vi "CalculerPolynome.vi"(6 "Résidu [in]":dbl, 8 "e3 [in]":dbl, 9 "Meilleure poly [in]":dbl[](array[numeric]), 10 "Y":dbl[](array[numeric]), 11 "X":dbl[](array[numeric])) -> (2 "Résidu [out]":dbl, 3 "Meilleur poly [out]":dbl[](array[numeric]))   [LabVIEW 2012]
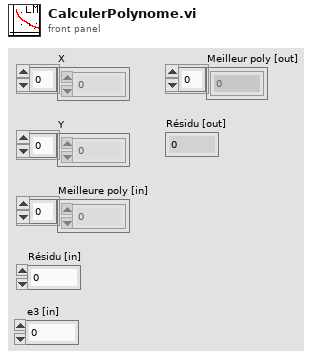
[diagram p1: front panel]
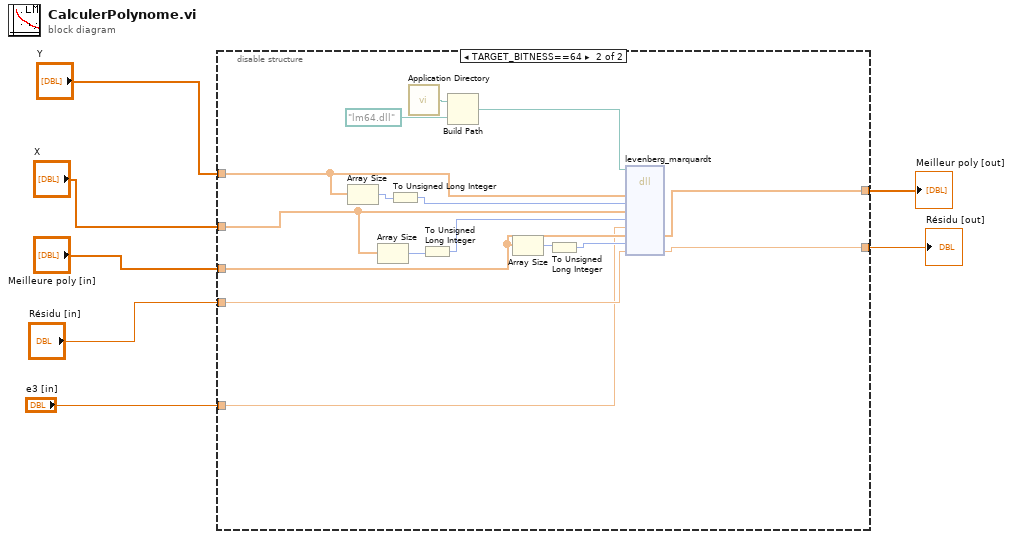
[diagram p0: block diagram]
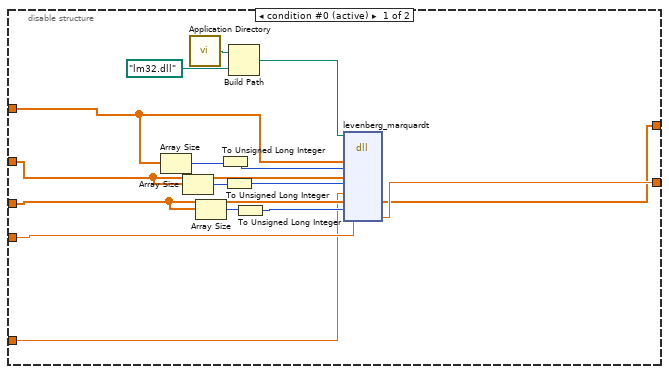
[diagram p2: hidden frame]
diagram:
  n1 = disable-structure shown="TARGET_BITNESS==64" {
    disable-tunnel: "X" -> [w14 w39]
    disable-tunnel: "Y" -> [w17 w38]
    disable-tunnel: "Meilleure poly [in]" -> [w20 w33]
    disable-tunnel: "Résidu [in]" -> [w23 w30]
    disable-tunnel: [w13 w29] -> w6
    disable-tunnel: [w12 w28] -> w7
    disable-tunnel: "e3 [in]" -> [w11 w27]
    frame condition #0 (active) {
      n2 = Array Size(array=w17) -> (size(s)=w18:i32)
      n3 = Array Size(array=w14) -> (size(s)=w15:i32)
      n4 = call <vilib>:"Application Directory.vi"() -> ("Application Directory"=w10:path)
      n5 = Array Size(array=w20) -> (size(s)=w21:i32)
      n6 = To Unsigned Long Integer(number=w18) -> (unsigned 32bit integer=w19:u32)
      n7 = To Unsigned Long Integer(number=w15) -> (unsigned 32bit integer=w16:u32)
      n8 = Build Path(base path=w10, name or relative path=path "lm32.dll" ("default name")) -> (appended path=w8:path)
      n9 = To Unsigned Long Integer(number=w21) -> (unsigned 32bit integer=w22:u32)
      n10 = dll-call lib="C:/Users/Damien/Documents/GitHub/TopView/lm32.dll" fn="levenberg_marquardt"(path in=w8, "yobs"=w17, "yobslength"=w19, "xobs"=w14, "xobslength"=w16, "e3"=w11, "polyptr"=w20, "numCoeffs"=w22, "e"=w23) -> ("polyptr"=w12:dbl[], "e"=w13:dbl)  [unwired: 9 in, 2 out]
    }
    frame condition #1 {
      n11 = Array Size(array=w38) -> (size(s)=w35:i32)
      n12 = Array Size(array=w39) -> (size(s)=w37:i32)
      n13 = To Unsigned Long Integer(number=w35) -> (unsigned 32bit integer=w34:u32)
      n14 = call <vilib>:"Application Directory.vi"() -> ("Application Directory"=w26:path)
      n15 = To Unsigned Long Integer(number=w37) -> (unsigned 32bit integer=w36:u32)
      n16 = Build Path(base path=w26, name or relative path=path "lm64.dll" ("default name")) -> (appended path=w24:path)
      n17 = Array Size(array=w33) -> (size(s)=w32:i32)
      n18 = To Unsigned Long Integer(number=w32) -> (unsigned 32bit integer=w31:u32)
      n19 = dll-call lib="C:/Users/MaxCorp/Documents/GitHub/TopView/lm64.dll" fn="levenberg_marquardt"(path in=w24, "yobs"=w38, "yobslength"=w34, "xobs"=w39, "xobslength"=w36, "e3"=w27, "polyptr"=w33, "numCoeffs"=w31, "e"=w30) -> ("polyptr"=w28:dbl[], "e"=w29:dbl)  [unwired: 9 in, 2 out]
    }
  }
  "Meilleur poly [out]" <- w7
  "Résidu [out]" <- w6
